vi "Initialize.vi"(0 "Rooms Manager Model in":refnum<class "Rooms Manager Model.lvclass">, 11 "error in (no error)":errorcluster) -> (4 "Rooms Manager Model out":refnum<class "Rooms Manager Model.lvclass">, 15 "error out":errorcluster)   [LabVIEW 2023, in "Rooms Manager Model.lvlib" / "Rooms Manager Model.lvclass"]
uses:
  Rooms Manager Model.lvclass
  C:/Program Files/National Instruments/LabVIEW 2023/vi.lib/ActorFramework/Actor/Actor.lvclass
  Rooms Manager UI/Rooms Manager UI/Rooms Manager UI.lvclass
  Rooms Manager Model Messages/Refresh Active Room Details Msg/Refresh Active Room Details Msg.lvclass
  C:/Users/bhaghyaraj/Trainings/NI Actor Framework/SDLC/Rooms Manager UI/Rooms Manager UI Messages/Refresh Active Room Details Msg/Refresh Active Room Details Msg.lvclass
  Rooms Manager Model Messages/Launch Guest Manager Msg/Launch Guest Manager Msg.lvclass
  C:/Users/bhaghyaraj/Trainings/NI Actor Framework/SDLC/Rooms Manager UI/Rooms Manager UI Messages/Launch Guest Manager Msg/Launch Guest Manager Msg.lvclass
  Rooms Manager UI/Rooms Manager UI/Rooms Manager UI.lvclass/Rooms Manager UI.ctl
  Rooms Manager Model.lvclass/Rooms Manager Model.ctl
  <vilib>/ActorFramework/Actor/Actor.lvclass
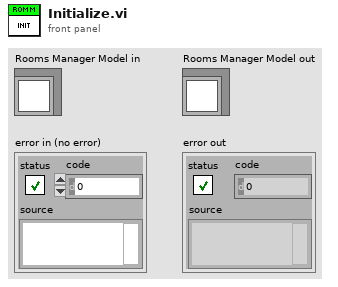
[diagram p1: front panel]
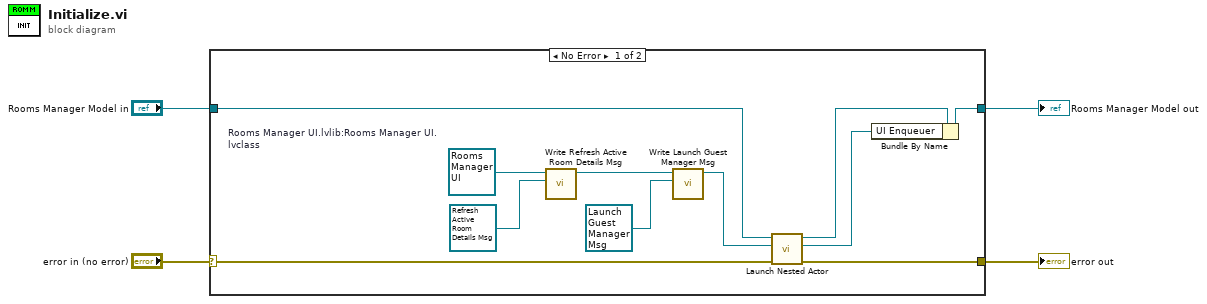
[diagram p0: block diagram]
diagram:
  n1 = case shown="No Error" "error in (no error)" {
    selector: "error in (no error)" -> [w10 w17]
    tunnel: [w15 w17] -> w2
    tunnel: [w12 w16] -> w1
    tunnel: "Rooms Manager Model in" -> [w14 w16]
    frame No Error {
      w9 = refnum<class "Rooms Manager UI.lvclass"> refnum  # Rooms Manager UI.lvlib:Rooms Manager UI.lvclass
      n2 = call "Write Refresh Active Room Details Msg.vi"("Rooms Manager UI.lvlib:Refresh Active Room Details Msg.lvclass"=refnum<class "Refresh Active Room Details Msg.lvclass"> refnum ("Rooms Manager Model.lvlib:Refresh Active Room Details Msg.lvclass"), "Rooms Manager UI in"=w9) -> ("Rooms Manager UI out"=w8:refnum<class "Rooms Manager UI.lvclass">)  [unwired: 9 in]
      n3 = call "Write Launch Guest Manager Msg.vi"("Rooms Manager UI.lvlib:Launch Guest Manager Msg.lvclass"=refnum<class "Launch Guest Manager Msg.lvclass"> refnum ("Rooms Manager Model.lvlib:Launch Guest Manager Msg.lvclass"), "Rooms Manager UI in"=w8) -> ("Rooms Manager UI out"=w6:refnum<class "Rooms Manager UI.lvclass">)  [unwired: 9 in]
      n4 = call <vilib>:"Launch Nested Actor.vi"("error in (no error)"=w10, "Nested Actor"=w6, "Caller Actor in"=w14) -> ("error out"=w15:errorcluster, "Nested Actor's Enqueuer"=w11:refnum<class "Message Enqueuer.lvclass">, "Caller Actor out"=w13:refnum<class "Rooms Manager Model.lvclass">)  [unwired: 6 in]
      n5 = Bundle By Name(cluster=w13, "UI Enqueuer"=w11) -> (w12:refnum<class "Rooms Manager Model.lvclass">)
    }
    frame Error {
    }
  }
  "error out" <- w2
  "Rooms Manager Model out" <- w1
